vi "closeTestStandEngine.vi"(8 "error in (no error)":errorcluster, 10 "Sequence File Ref":refnum<k7>, 11 "Engine Reference":refnum<k7>) -> (0 "error out":errorcluster)   [LabVIEW 2010]
panel:
  out "ReleaseSequenceFileEx":bool
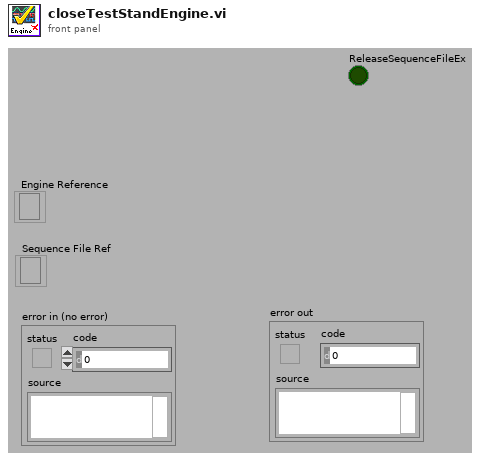
[diagram p1: front panel]
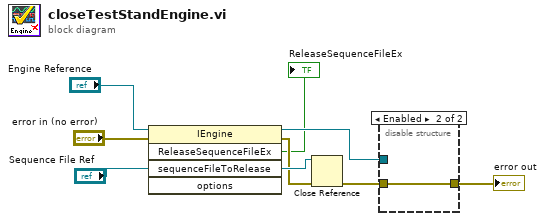
[diagram p0: block diagram]
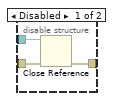
[diagram p2: hidden frame]
diagram:
  n1 = invoke class="IEngine" method="ReleaseSequenceFileEx"(reference="Engine Reference", error in="error in (no error)", "sequenceFileToRelease"="Sequence File Ref") -> (reference out=w5:refnum<k7>, error out=w3:errorcluster, "ReleaseSequenceFileEx"=→"ReleaseSequenceFileEx":bool)  [unwired: 2 in, 2 out]
  n2 = Close Reference(reference="Sequence File Ref", error in (no error)=w3) -> (error out=w8:errorcluster)
  n3 = disable-structure shown="Enabled" {
    disable-tunnel: w8 -> [w11 w12]
    disable-tunnel: w5 -> [w10 _]
    disable-tunnel: [w9 w12] -> w2
    frame Disabled {
      n4 = Close Reference(reference=w10, error in (no error)=w11) -> (error out=w9:errorcluster)
    }
    frame Enabled {
    }
  }
  "error out" <- w2
